vi "test Acyclic Frame Address Pairs In Log.vi"(8 "error in (no error)":errorcluster, 11 "TestCase in":refnum<class "Logging Loopback.lvclass">) -> (0 "error out":errorcluster, 3 "TestCase out":refnum<class "Logging Loopback.lvclass">)   [LabVIEW 2020, in "Logging Loopback.lvclass"]
uses:
  Logging Loopback.lvclass
  Logging Loopback.lvclass/Logging Loopback.ctl
  6070ecc1-7a7f-4aba-84f3-8f274e3c644e.vi
  <vilib>/WebDAVClient/Advanced/Get Buffer.vi
  <vilib>/addons/_JKI Toolkits/VI Tester/TestCase.llb/TestCase.lvclass
  <vilib>/WebDAVClient/NI_WebDAV.lvlib
  C:/Program Files (x86)/National Instruments/LabVIEW 2020/vi.lib/addons/_JKI Toolkits/VI Tester/TestCase.llb/TestCase.lvclass
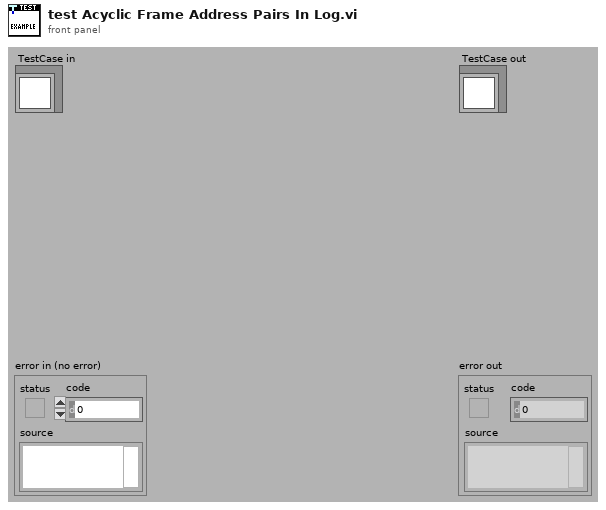
[diagram p1: front panel]
types:
  T1 = typedef "NI_WebDAV.lvlib/SessionHandle.ctl" = refnum<k1>
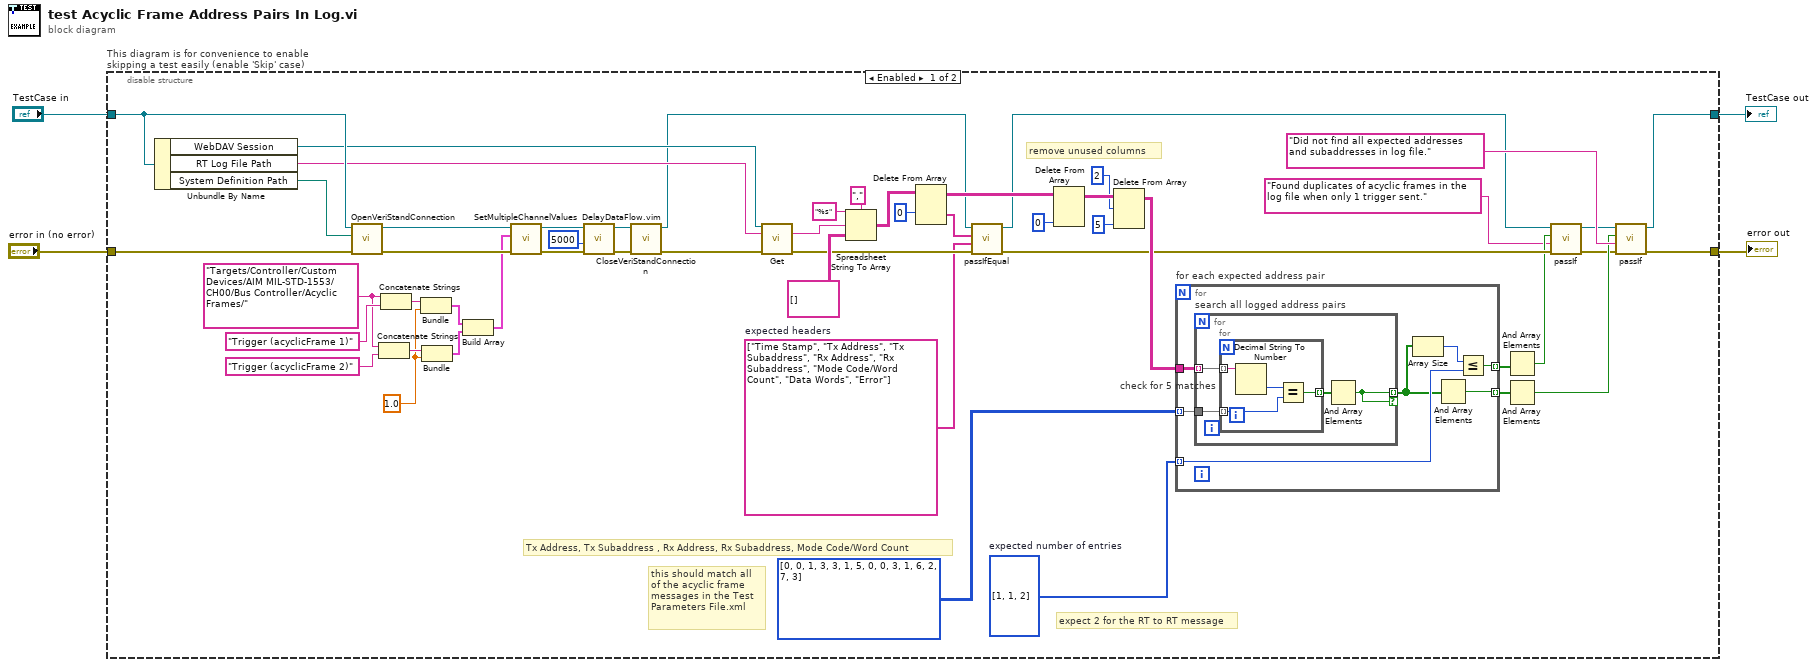
[diagram p0: block diagram]
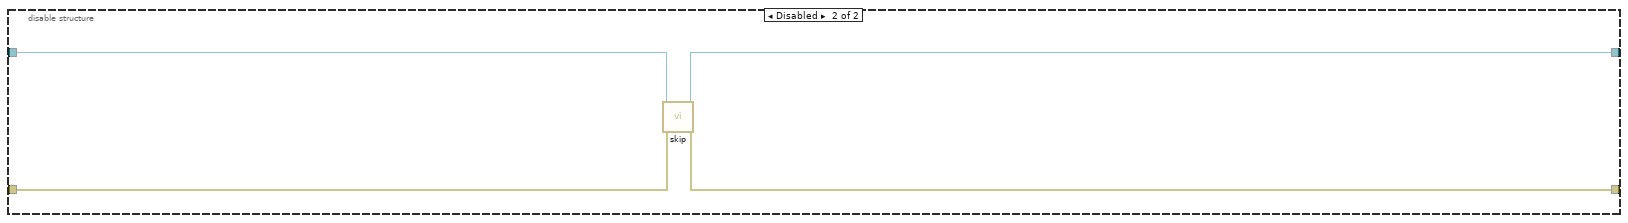
[diagram p2: hidden frame]
diagram:
  n1 = disable-structure "This diagram is for convenience to enable skipping a test easily (enable 'Skip' case)" shown="Enabled" {
    disable-tunnel: "TestCase in" -> [w52 w74]
    disable-tunnel: [w41 w72] -> w1
    disable-tunnel: [w42 w73] -> w3
    disable-tunnel: "error in (no error)" -> [w55 w71]
    frame Enabled {
      w5 = i32[] [1, 1, 2]  # expected number of entries
      w8 = 1.0
      w11 = "Targets/Controller/Custom Devices/AIM MIL-STD-1553/CH00/Bus Controller/Acyclic Frames/" ("base name for channel aliases")
      w26 = string[] ["Time Stamp", "Tx Address", "Tx Subaddress", "Rx Address", "Rx Subaddress", "Mode Code/Word Count", "Data Words", "Error"]  # expected headers
      # "expect 2 for the RT to RT message"
      # "remove unused columns"
      # "this should match all of the acyclic frame messages in the Test Parameters File.xml"
      # "Tx Address, Tx Subaddress , Rx Address, Rx Subaddress, Mode Code/Word Count"
      n2 = Unbundle By Name(w52) -> ("WebDAV Session"=w48:T1, "RT Log File Path"=w47:string, "System Definition Path"=w53:path)
      n3 = call-dynamic "OpenVeriStandConnection.vi"("error in (no error)"=w55, "System Definition File"=w53, "VeriStand Test Case in"=w52) -> ("error out"=w54:errorcluster, "VeriStand Test Case out"=w23:refnum<class "Logging Loopback.lvclass">)  [unwired: 6 in, 1 out]
      n4 = Concatenate Strings(w11, "Trigger (acyclicFrame 2)" ("base name for channel aliases")) -> (w9:string)
      n5 = Concatenate Strings(w11, "Trigger (acyclicFrame 1)" ("base name for channel aliases")) -> (w19:string)
      n6 = Bundle(w19, w8) -> (w20:cluster{string, dbl})  [unwired: 1 in]
      n7 = Bundle(w9, w8) -> (w6:cluster{string, dbl})  [unwired: 1 in]
      n8 = Build Array(w20, w6) -> (w21:cluster{string, dbl}[])
      n9 = call-dynamic "SetMultipleChannelValues.vi"("error in (no error)"=w54, "Channel Key Value Pairs in"=w21, "VeriStandTestCase in"=w23) -> ("error out"=w24:errorcluster, "VeriStandTestCase out"=w22:refnum<class "Logging Loopback.lvclass">)  [unwired: 7 in]
      n10 = call "DelayDataFlow.vim"("value in"=w24, "milliseconds to wait"=u32 5000) -> ("value out"=w51:errorcluster)  [unwired: 2 in, 1 out]
      n11 = call-dynamic "CloseVeriStandConnection.vi"("error in (no error)"=w51, "VeriStand Test Case in"=w22) -> ("error out"=w49:errorcluster, "VeriStand Test Case out"=w28:refnum<class "Logging Loopback.lvclass">)  [unwired: 8 in]
      n12 = call-poly <vilib>:"Get.vi"("session handle"=w48, "relative uri"=w47, "error in (no error)"=w49) -> ("data"=w46:string, "error out"=w29:errorcluster)  [unwired: 10 in, 1 out]
      n13 = Spreadsheet String To Array(delimiter (Tab)=",", format string="%s", spreadsheet string=w46, array type (2D Dbl)=string[][] []) -> (array=w31:string[][])
      n14 = Delete From Array(array=w31, index (row)=0) -> (deleted portion=w27:string[], array with subset deleted=w30:string[][])  [unwired: 2 in]
      n15 = call-dynamic "passIfEqual.vi"("error in (no error)"=w29, "y"=w26, "x"=w27, "TestCase in"=w28) -> ("error out"=w18:errorcluster, "TestCase out"=w17:refnum<class "Logging Loopback.lvclass">)  [unwired: 6 in]
      n16 = Delete From Array(array=w30, index (col)=0 ("disabled index (col)")) -> (array with subset deleted=w37:string[][])  [unwired: 2 in, 1 out]
      n17 = Delete From Array(array=w37, length=2, index (col)=5 ("disabled index (col)")) -> (array with subset deleted=w35:string[][])  [unwired: 1 in, 1 out]
      n18 = for "for each expected address pair" {
        tunnel: w35 -> [w62]
        tunnel: i32[][] [[0, 0, 1, 3, 3], [1, 5, 0, 0, 3], [1, 6, 2, 7, 3]] -> [w61] mode=indexing
        tunnel: [w56] -> w33 mode=indexing
        tunnel: [w59] -> w7 mode=indexing
        tunnel: w5 -> [w58] mode=indexing
        n19 = for "search all logged address pairs" {
          tunnel: w62 -> [w66] mode=indexing
          tunnel: w61 -> [w65]
          tunnel: [w63] -> w57 mode=indexing if=w63
          n20 = for "check for 5 matches" {
            tunnel: w66 -> [w70] mode=indexing
            tunnel: w65 -> [w68] mode=indexing
            tunnel: [w67] -> w64 mode=indexing
            n21 = Decimal String To Number(string=w70) -> (number=w69:i32)  [unwired: 2 in, 1 out]
            n22 = Equal?(x=w69, y=w68) -> (x = y?=w67:bool)
          }
          n23 = And Array Elements(Boolean array=w64) -> (logical AND=w63:bool)
        }
        n24 = Array Size(array=w57) -> (size(s)=w60:i32)
        n25 = And Array Elements(Boolean array=w57) -> (logical AND=w56:bool)
        n26 = Less Or Equal?(x=w60, y=w58) -> (x <= y?=w59:bool)
      }
      n27 = And Array Elements(Boolean array=w7) -> (logical AND=w14:bool)
      n28 = And Array Elements(Boolean array=w33) -> (logical AND=w32:bool)
      n29 = call-dynamic "passIf.vi"("error in (no error)"=w18, "message (\"\")"="Found duplicates of acyclic frames in the log file when only 1 trigger sent." ("message (\"\")"), "pass"=w14, "TestCase in"=w17) -> ("error out"=w15:errorcluster, "TestCase out"=w16:refnum<class "Logging Loopback.lvclass">)  [unwired: 6 in]
      n30 = call-dynamic "passIf.vi"("error in (no error)"=w15, "message (\"\")"="Did not find all expected addresses and subaddresses in log file." ("message (\"\")"), "pass"=w32, "TestCase in"=w16) -> ("error out"=w42:errorcluster, "TestCase out"=w41:refnum<class "Logging Loopback.lvclass">)  [unwired: 6 in]
    }
    frame Disabled {
      # "skip test result while test is under development"
      n31 = call <vilib>:"skip.vi"("error in (no error)"=w71, "TestCase in"=w74) -> ("error out"=w73:errorcluster, "TestCase out"=w72:refnum<class "Logging Loopback.lvclass">)  [unwired: 8 in]
    }
  }
  "error out" <- w3
  "TestCase out" <- w1
